vi "Conv to num.vi"(8 "Column":i32, 9 "Row":i32, 11 "Array":string[][](array[string])) -> (2 "result string":string)   [LabVIEW 2014]
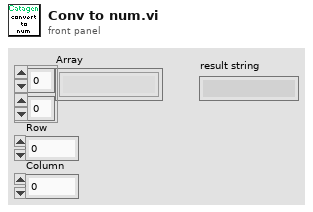
[diagram p1: front panel]
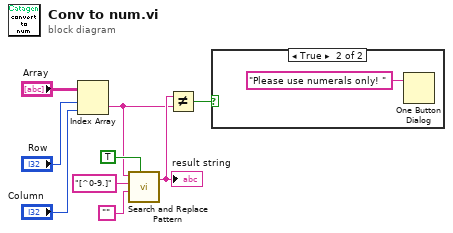
[diagram p0: block diagram]
diagram:
  n1 = Index Array(array="Array", index (row)="Row", index (col)="Column") -> (element=w1:string)
  n2 = call <vilib>:"Search and Replace Pattern.vi"("string"=w1, "regular expression (\"\")"="[^0-9.]" ("format string"), "replace string (\"\")"="", "replace all? (F)"=TRUE) -> ("result string"=w3:string)  [unwired: 1 in, 1 out]
  "result string" <- w3
  n3 = Not Equal?(x=w3, y=w1) -> (x != y?=w2:bool)
  n4 = case shown="True" w2 {
    frame False {
    }
    frame True {
      n5 = One Button Dialog(message="Please use numerals only! ") -> ()  [unwired: 1 in, 1 out]
    }
  }
